vi "Version 1_Write Batch SetPoint.vi"(7 "Unit ID (A)":string="A", 8 "error in":errorcluster, 9 "Batch SetPoint":dbl, 11 "VISA Session In":refnum<visa-resource-name>="Alicat") -> (0 "error out":errorcluster, 3 "VISA Session Out":refnum<visa-resource-name>)   [LabVIEW 2014]
doc: "Writes a batch setpoint into an Alicat device. ONLY AVAILABLE FOR R22 BOARDS AND ABOVE (run \"Legacy Detector.vi\" to determine board revision), provided that the unit is a controller with totalizer functionality and a firmware version of at least 4v33."
uses:
  <vilib>/Instr/_visa.llb/VISA Flush IO Buffer Mask.ctl
panel:
  # "ONLY AVAILABLE FOR R22 BOARDS AND ABOVE\n(provided it is a controller with totalizer and at least firmware 4v33)"
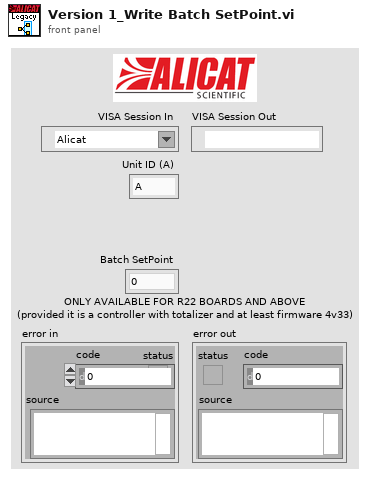
[diagram p1: front panel]
types:
  T1 = typedef "VISA Flush IO Buffer Mask.ctl" = u16
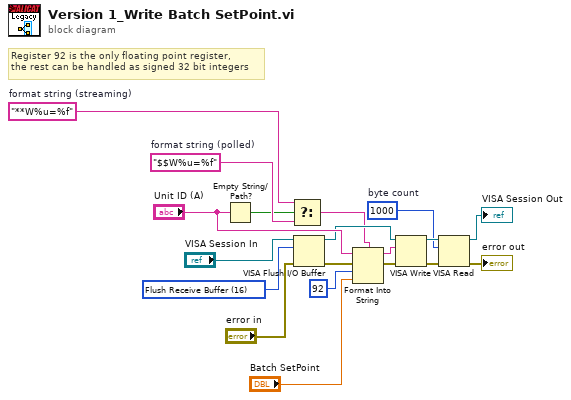
[diagram p0: block diagram]
diagram:
  w2 = "**W%u=%f"  # format string (streaming)
  w4 = "$$W%u=%f"  # format string (polled)
  w11 = T1 16 items=["Flush Receive Buffer"=16, "Write Transmit Buffer to Device"=32, "Flush Receive Buffer (No I/O)"=64, "Flush Transmit Buffer"=128] ("Mask")
  w9 = u32 1000  # byte count
  # "Register 92 is the only floating point register, \nthe rest can be handled as signed 32 bit integers"
  n1 = Empty String/Path?(string/path="Unit ID (A)") -> (empty?=w3:bool)
  n2 = Select(t=w2, s=w3, f=w4) -> (s? t:f=w1:string)
  n3 = VISA Flush I/O Buffer(VISA resource name="VISA Session In", mask (16)=w11, error in (no error)="error in") -> (VISA resource name out=w12:refnum<visa-resource-name>, error out=w7:errorcluster)
  n4 = Format Into String(format string=w1, initial string="Unit ID (A)", error in=w7, u16 92 ("Register address"), "Batch SetPoint") -> (resulting string=w8:string, error out=w6:errorcluster)
  n5 = VISA Write(VISA resource name=w12, write buffer=w8, error in (no error)=w6) -> (VISA resource name out=w10:refnum<visa-resource-name>, error out=w13:errorcluster)  [unwired: 1 out]
  n6 = VISA Read(VISA resource name=w10, byte count=w9, error in (no error)=w13) -> (VISA resource name out=→"VISA Session Out":refnum<visa-resource-name>, error out=→"error out":errorcluster)  [unwired: 2 out]
